vi "Neighbors.vi"(10 "Size":i32, 11 "index":i32) -> (3 "Neighbors":enum16{"None", "Both", "Lower", "Upper"}(ring))   [LabVIEW 2014]
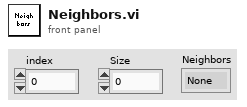
[diagram p1: front panel]
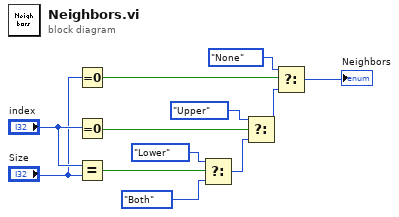
[diagram p0: block diagram]
diagram:
  n1 = Equal To 0?(x="Size") -> (x = 0?=w8:bool)
  n2 = Equal To 0?(x="index") -> (x = 0?=w11:bool)
  n3 = Equal?(x="index", y="Size") -> (x = y?=w10:bool)
  n4 = Select(t=enum16{"None", "Both", "Lower", "Upper"}."Lower", s=w10, f=enum16{"None", "Both", "Lower", "Upper"}."Both") -> (s? t:f=w7:enum16{"None", "Both", "Lower", "Upper"})
  n5 = Select(t=enum16{"None", "Both", "Lower", "Upper"}."Upper", s=w11, f=w7) -> (s? t:f=w2:enum16{"None", "Both", "Lower", "Upper"})
  n6 = Select(t=enum16{"None", "Both", "Lower", "Upper"}."None", s=w8, f=w2) -> (s? t:f=→"Neighbors":enum16{"None", "Both", "Lower", "Upper"})
